vi "getValuesDbl.vi"(8 "error in":errorcluster, 9 "timeout in ms (-1)":i32=100, 11 "notifiers in":refnum<notifier>[](array[refnum])) -> (0 "error out":errorcluster, 2 "notifier values":string[](array[string]), 3 "notifier names":string[](array[string]))   [LabVIEW 2013]
doc: "Takes an array of notifiers and returns two arrays containing the name and value of each notifier. All values have been flattened to strings.\nNotifier value must be a double.\n\nKaitlin Gallagher\n3/4/14"
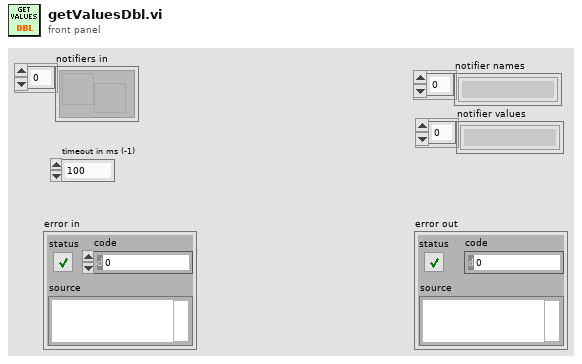
[diagram p1: front panel]
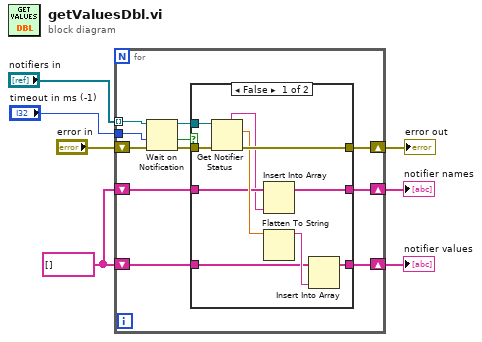
[diagram p0: block diagram]
diagram:
  w3 = string[] [] ("notifier names 2")
  n1 = for {
    tunnel: "notifiers in" -> [w17] mode=indexing
    shift-right: [w18] -> w5
    shift-left: "error in" -> [w15]
    tunnel: "timeout in ms (-1)" -> [w13]
    shift-right: [w10] -> w2
    shift-left: w3 -> [w11]
    shift-right: [w8] -> w1
    shift-left: w3 -> [w9]
    n2 = Wait on Notification(notifier=w17, timeout in ms (-1)=w13, error in (no error)=w15) -> (notifier out=w16:refnum<notifier>, timed out?=w12:bool, error out=w14:errorcluster)  [unwired: 1 in, 1 out]
    n3 = case shown="False" w12 {
      tunnel: [w28 w31] -> w18
      tunnel: w16 -> [w26 _]
      tunnel: w14 -> [w25 w31]
      tunnel: w11 -> [w24 w30]
      tunnel: [w23 w30] -> w10
      tunnel: w9 -> [w20 w29]
      tunnel: [w19 w29] -> w8
      frame False {
        n4 = Get Notifier Status(notifier=w26, error in (no error)=w25) -> (notifier name=w22:string, current notification=w27:dbl, error out=w28:errorcluster)  [unwired: 2 out]
        n5 = Insert Into Array(array=w24, new element=w22) -> (w23:string[])  [unwired: 1 in]
        n6 = Flatten To String(anything=w27) -> (data string=w21:string)  [unwired: 3 in, 2 out]
        n7 = Insert Into Array(array=w20, new element=w21) -> (w19:string[])  [unwired: 1 in]
      }
      frame True {
      }
    }
  }
  "error out" <- w5
  "notifier names" <- w2
  "notifier values" <- w1
